vi "Create Enum Setter.vi"(7 "RPC Message Name":string, 8 "error in (no error)":errorcluster, 11 "RPC Messages Folder (ProjectItem) in":refnum<vi>) -> (0 "error out":errorcluster, 2 "Message Setter out":refnum<vi>, 3 "RPC Messages Folder (ProjectItem) out":refnum<vi>)   [LabVIEW 2019, in "gRPC Template Creation Utility.lvlib"]
uses:
  gRPC Template Creation Utility.lvlib
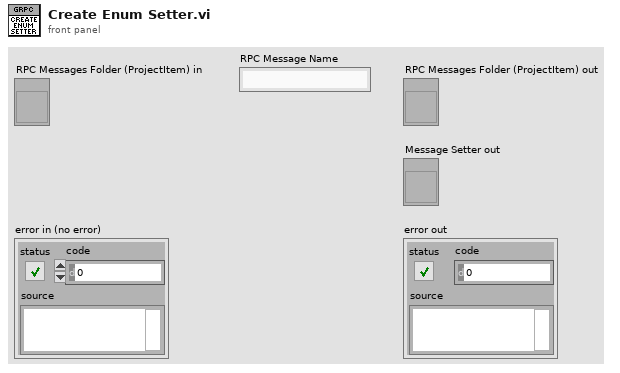
[diagram p1: front panel]
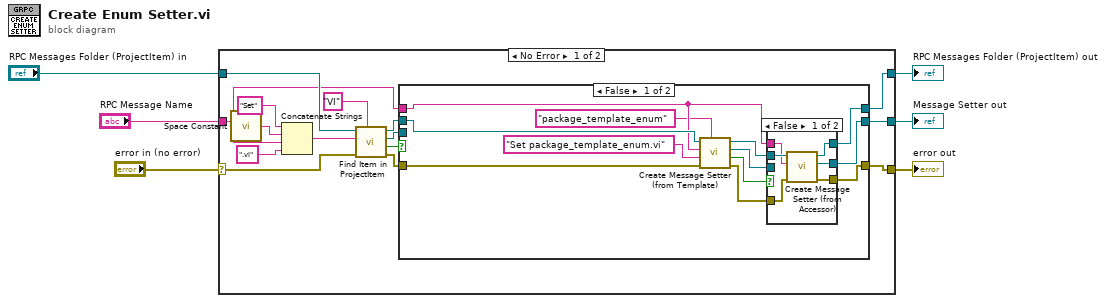
[diagram p0: block diagram]
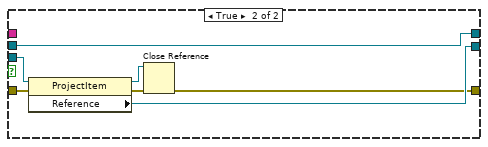
[diagram p3: hidden frame]
diagram:
  n1 = case shown="No Error" "error in (no error)" {
    selector: "error in (no error)" -> [w15 w51]
    tunnel: [w9 w50] -> w6
    tunnel: [w7 w51] -> w5
    tunnel: "RPC Messages Folder (ProjectItem) in" -> [w20 w50]
    tunnel: "RPC Message Name" -> [w11 _]
    tunnel: [w8 _] -> w1
    frame No Error {
      n2 = call <vilib>:"Space Constant.vi"() -> ("String"=w18:string)
      n3 = Concatenate Strings("Set" ("string"), w18, w11, ".vi" ("string")) -> (w16:string)
      n4 = call "Find Item in ProjectItem.vi"("Item Type"="VI", "error in (no error)"=w15, "Name"=w16, "ProjectItem in"=w20) -> ("error out"=w10:errorcluster, "Found ?"=w13:bool, "Item Refnum out"=w12:refnum<vi>, "ProjectItem out"=w14:refnum<vi>)  [unwired: 4 in]
      n5 = case shown="False" w13 {
        tunnel: [w32 w48] -> w8
        tunnel: [w33 w47] -> w9
        tunnel: w10 -> [w29 w43]
        tunnel: [w31 w44] -> w7
        tunnel: w14 -> [w30 w47]
        tunnel: w12 -> [_ w49]
        tunnel: w11 -> [w24 _]
        frame False {
          n6 = call "Create Message Setter (from Template).vi"("replace string in template"="package_template_enum", "error in (no error)"=w29, "template VI name"="Set package_template_enum.vi", "RPC Message Name"=w24, "RPC Messages Folder (ProjectItem) in"=w30) -> ("error out"=w25:errorcluster, "Created?"=w26:bool, "VI out"=w27:refnum<vi>, "RPC Messages Folder (ProjectItem) out"=w28:refnum<vi>)  [unwired: 3 in]
          n7 = case shown="False" w26 {
            tunnel: w25 -> [w38 w41]
            tunnel: w28 -> [w39 w42]
            tunnel: w27 -> [_ w40]
            tunnel: [w36 w42] -> w33
            tunnel: [w34 w41] -> w31
            tunnel: [w35 w40] -> w32
            tunnel: w24 -> [w37 _]
            frame False {
              n8 = call "Create Message Setter (from Accessor).vi"("error in (no error)"=w38, "RPC Message Name"=w37, "RPC Messages Folder (ProjectItem) in"=w39) -> ("error out"=w34:errorcluster, "Getter VI out"=w35:refnum<vi>, "RPC Messages Folder (ProjectItem) out"=w36:refnum<vi>)  [unwired: 5 in, 1 out]
            }
            frame True {
            }
          }
        }
        frame True {
          n9 = property class="ProjectItem"(reference=w49, error in=w43) -> (reference out=w45:refnum<vi>, error out=w46:errorcluster, "Reference"=w48:refnum<vi>)
          n10 = Close Reference(reference=w45, error in (no error)=w46) -> (error out=w44:errorcluster)
        }
      }
    }
    frame Error {
    }
  }
  "error out" <- w5
  "Message Setter out" <- w1
  "RPC Messages Folder (ProjectItem) out" <- w6
